vi "HW_Setup_2.vi"(8 "error in":errorcluster, 9 "Close port? (F)":bool, 10 "Target FPS":T1, 11 "VISA resource name in":refnum<visa-resource-name>="Tracker") -> (0 "error out":errorcluster, 1 "Sync mode status":string, 2 "HW information":string, 3 "VISA resource name out":refnum<visa-resource-name>, 4 "Instrument OK?":bool, 5 "Sync capability":u8, 7 "FPS status":i32=80)   [LabVIEW 2018]
uses:
  Controls/CTL_Acquisition_speed_selector.ctl
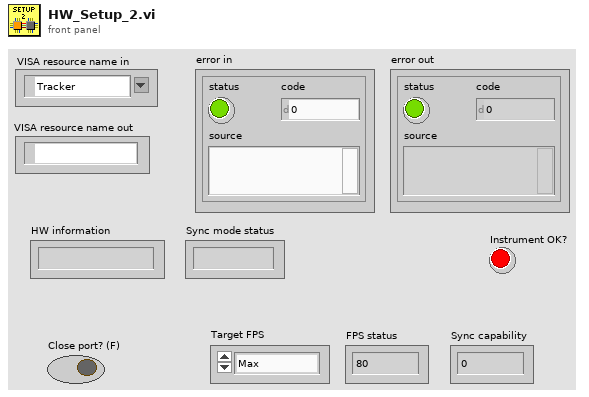
[diagram p1: front panel]
types:
  T1 = typedef "CTL_Acquisition_speed_selector.ctl" = enum16{"Max", "High stability", "Eco"}
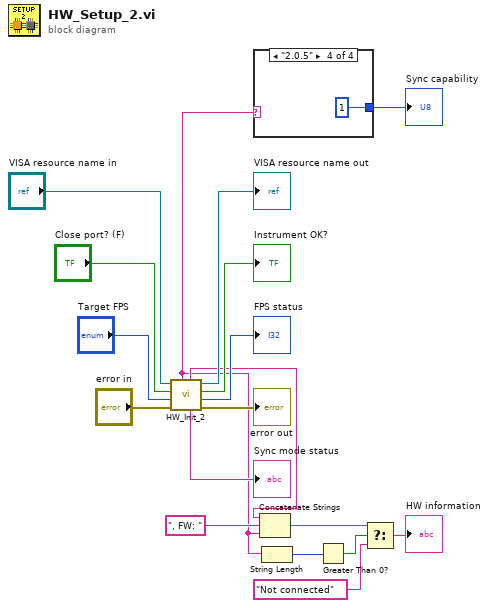
[diagram p0: block diagram]
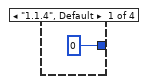
[diagram p2: hidden frame]
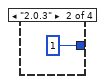
[diagram p3: hidden frame]
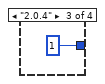
[diagram p4: hidden frame]
diagram:
  n1 = call "HW_Init_2.vi"("error in"="error in", "Target FPS"="Target FPS", "Close port? (F)"="Close port? (F)", "VISA resource name"="VISA resource name in") -> ("error out"=→"error out":errorcluster, "FPS status"=→"FPS status":i32, "Instrument OK?"=→"Instrument OK?":bool, "VISA resource name out"=→"VISA resource name out":refnum<visa-resource-name>, "Sync mode status"=→"Sync mode status":string, "Sensor board size"=w4:string, "FW version information"=w2:string)  [unwired: 1 in]
  n2 = case shown="\"2.0.5\"" w2 {
    tunnel: [u8 0 u8 1 u8 1 u8 1] -> w1
    frame "1.1.4", Default {
    }
    frame "2.0.3" {
    }
    frame "2.0.4" {
    }
    frame "2.0.5" {
    }
  }
  "Sync capability" <- w1
  n3 = Concatenate Strings(w4, ", FW: " ("string"), w2) -> (w7:string)
  n4 = String Length(string=w2) -> (length=w5:i32)
  n5 = Greater Than 0?(x=w5) -> (x > 0?=w8:bool)
  n6 = Select(t=w7, s=w8, f="Not connected") -> (s? t:f=→"HW information":string)
